vi "Write Serializaton Binder Base Class Then Read - Returns Default Serialization Binder.vi"() -> ()   [LabVIEW 2017, in "Generic Object Serializer Tests.lvlib" / "Serialization Binder.lvlib"]
uses:
  Serialization Binder.lvlib
  Generic Object Serializer/Generic Object Serializer.lvclass
  Default Serialization Binder/Default Serialization Binder.lvclass
  C:/Users/de200256/Code/logmanoriginal/jsontext-object-serialization/Serialization Binder/Serialization Binder.lvclass
  Serialization Binder/Serialization Binder.lvclass
  Generic Object Serializer/Generic Object Serializer.lvclass/Generic Object Serializer.ctl
  Generic Object Serializer/Write Serialization Binder.vi
  Generic Object Serializer/Read Serialization Binder.vi
  <vilib>/addons/_JKI Toolkits/Caraya/classes/Assert/Assert.lvclass
  <vilib>/addons/_JKI Toolkits/Caraya/classes/Test/Test.lvclass
panel:
  out "error out":errorcluster
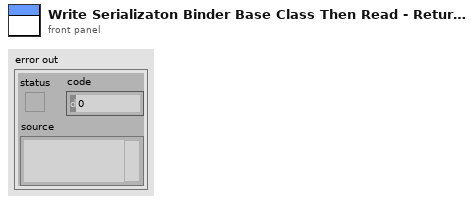
[diagram p1: front panel]
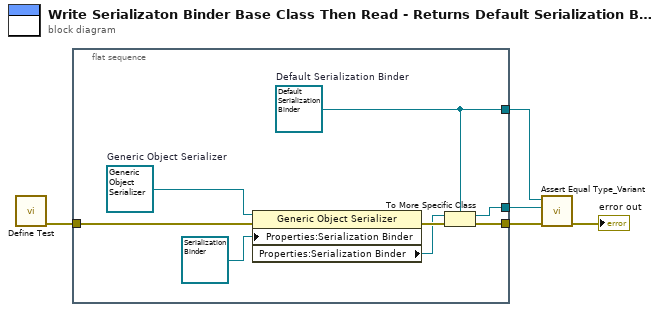
[diagram p0: block diagram]
diagram:
  n1 = call <vilib>:"Define Test.vi"() -> ("error out"=w3:errorcluster)  [unwired: 11 in]
  n2 = flat-sequence {
    tunnel: [w8] -> w5
    tunnel: [w7] -> w4
    tunnel: w3 -> [w12]
    tunnel: [w10] -> w2
    frame #0 {
      w7 = refnum<class "Default Serialization Binder.lvclass"> refnum  # Default Serialization Binder
      w13 = refnum<class "Generic Object Serializer.lvclass"> refnum  # Generic Object Serializer
      n3 = property class="Generic Object Serializer"(reference=w13, error in=w12, "Properties:Serialization Binder"=refnum<class "Serialization Binder.lvclass"> refnum ("Serialization Binder")) -> (error out=w11:errorcluster, "Properties:Serialization Binder"=w9:refnum<class "Serialization Binder.lvclass">)  [unwired: 1 out]
      n4 = To More Specific Class(target class=w7, reference=w9, error in=w11) -> (specific class reference=w8:refnum<class "Default Serialization Binder.lvclass">, error out=w10:errorcluster)
    }
  }
  n5 = call <vilib>:"Assert Equal Type_Variant.vi"("error in (no error)"=w2, "Y"=w5, "X"=w4) -> ("error out"=→"error out":errorcluster)  [unwired: 8 in]
